vi "Transient Amb.vi"() -> ()   [LabVIEW 2015]
uses:
  <vilib>/Platform/TimedLoop/XDataNode/timing_clust.ctl
  <vilib>/Platform/TimedLoop/XDataNode/nitl_modes.ctl
  <vilib>/Platform/TimedLoop/XDataNode/wakeup.ctl
  <vilib>/DAQmx/read.llb/DAQmx Read (Analog DBL 1Chan 1Samp).vi
  <vilib>/DAQmx/read.llb/DAQmx Read (Analog 1D DBL NChan 1Samp).vi
  <vilib>/DAQmx/create/channels.llb/DAQmx Create Channel (AI-Voltage-Basic).vi
  <vilib>/DAQmx/miscellaneous.llb/DAQmx Fill In Error Info.vi
  <vilib>/Platform/TimedLoop/XDataNode/XDataNode.xnode
  Program Files/neMESYS_SDK/neMESYS LabVIEW Kit/neMESYS LabVIEW Integration Kit.lvlib
  <vilib>/Platform/TimedLoop/XDataNode/XDNodeRunTimeDep.lvlib
  Conor/Temp CN7500/Omega CN7500/Omega CN7500.lvlib
panel:
  out "Iteration Number":dbl
  in  "Ramp Temp":bool
  in  "Temp Decrease per Minute":dbl
  in  "Start Temp":dbl
  in  "Minutes at Start Conditions":dbl
  in  "Ramp Flow":bool
  in  "Flow Decrease per Minute":dbl
  in  "Start Flowrate":dbl
  in  "Flowrate 4":dbl
  in  "Flowrate 3":dbl
  in  "Flowrate 2":dbl
  in  "Flowrate 1":dbl
  in  "Temp Set Point":dbl
  out "Liquid Inlet Pressure (bar g)":dbl
  in  "Liquid P sensor Terminal Configuration":i32(ring)=-1 items=["default"=-1, "RSE"=10083, "NRSE"=10078, "Differential"=10106, "Pseudodifferential"=12529]
  in  "Liquid P sensor Physical Channel":tag="Dev1/ai0"
  in  "Safety or Emergency Syringe Control":bool
  out "Total Flowrate (uL/min)":dbl
  out "Gas Back Pressure (barg)":dbl
  in  "Shut down in empty?\nLeft off, right on":bool
  in  "Clear":bool
  out "Safety Shut Down Pressure (barg)":dbl
  out "Calculated Pressure":dbl[](graph)
  out "Safety Shut Down Temp":dbl
  out "Actual Temp (oC)":dbl
  out "Temperature":dynamicdata(graph)
  out "Temp Set Point (oC)":dbl
  in  "Stop everything":bool
  in  "Refill 4":bool
  in  "Refill 3":bool
  in  "Refill 2":bool
  in  "Refill 1":bool
  in  "Empty 4":bool
  in  "Empty 3":bool
  in  "Empty 2":bool
  in  "Empty 1":bool
  in  "Calibrate 4":bool
  in  "Calibrate 3":bool
  in  "Calibrate 2":bool
  in  "Calibrate 1":bool
  in  "Stop Dose 4":bool
  in  "Stop Dose 3":bool
  in  "Stop Dose 2":bool
  in  "Stop Dose 1":bool
  out "Syringe Level 4":dbl(slide) scale=0.0..5500.0
  out "Syringe Level 3":dbl(slide) scale=0.0..5500.0
  out "Syringe Level 2":dbl(slide) scale=0.0..5500.0
  out "Syringe Level 1":dbl(slide) scale=0.0..5500.0
  out "Flowrate 4 Ethanol":dbl
  out "Flowrate 3 Acid":dbl
  out "Flowrate 2 High":dbl
  out "Flowrate 1 Low":dbl
  # "Safety (start and end)"
  # "Current Conditions"
  # "(uL/min)"
  # "Coerced to nearest possible"
  # "If either ramps are off you need to manually enter the constant flowrate or temperature in the \nbottom sections"
  # "This code just uses 2 syringes\nThe ones at the right hand side"
  # "Emergency Syringe Control Below"
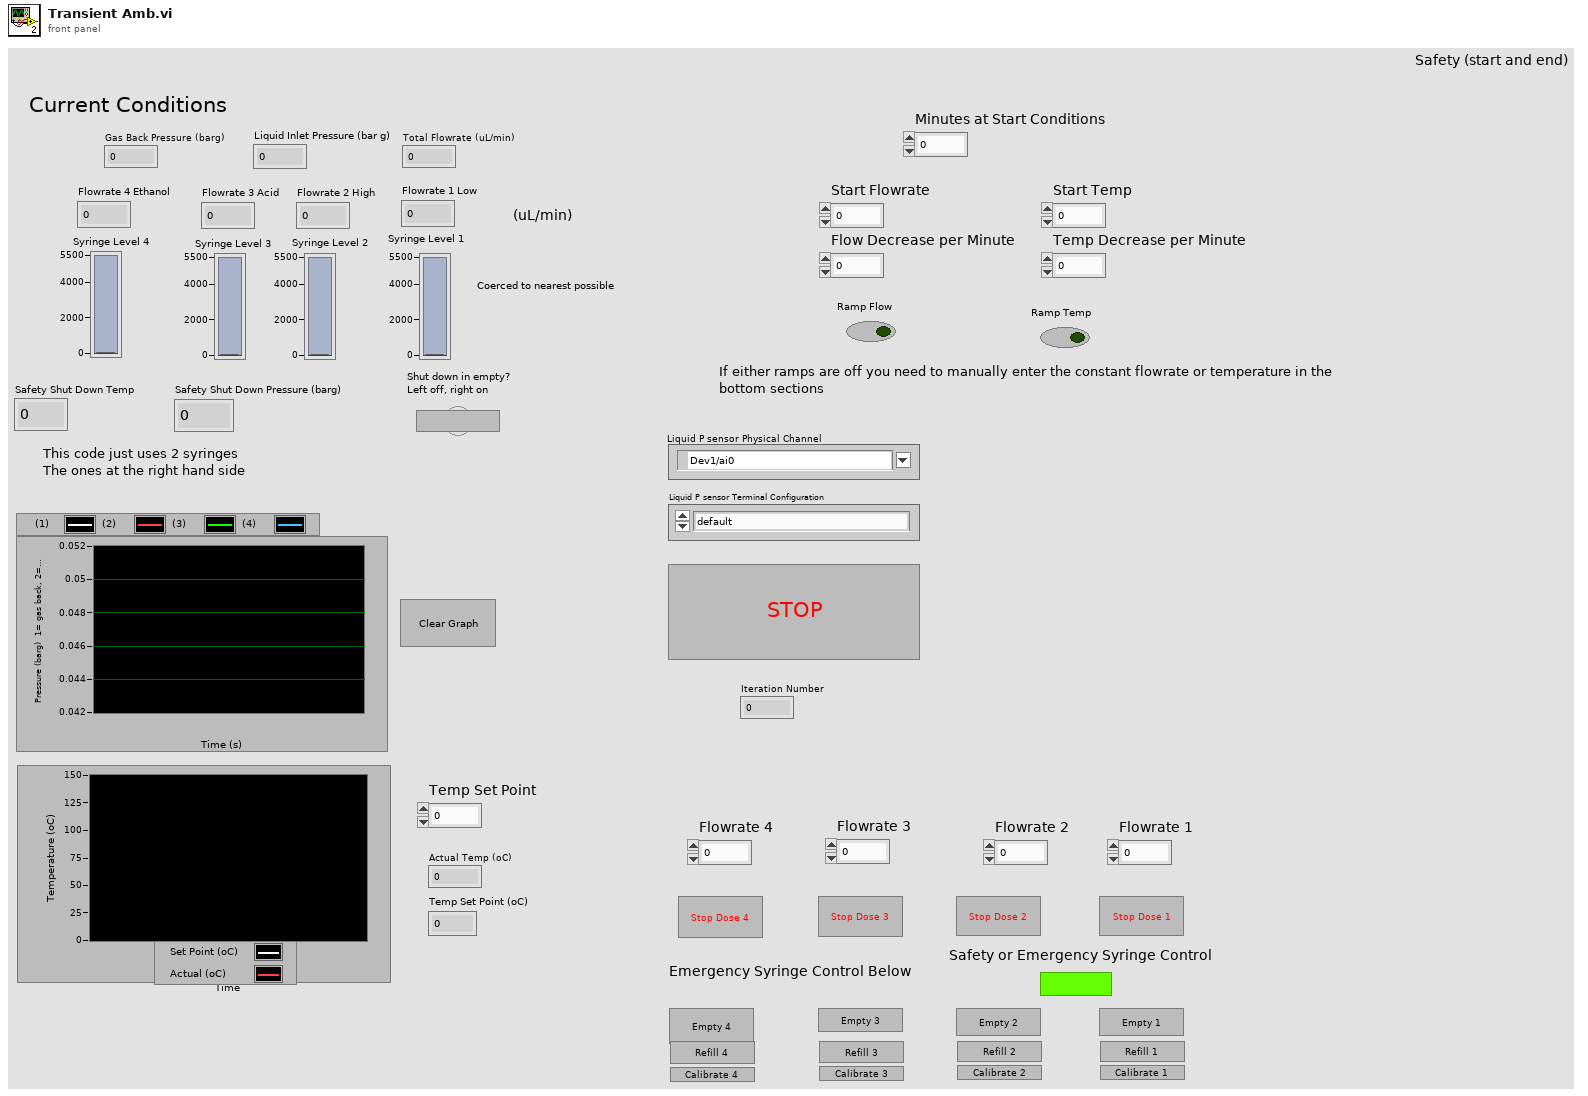
[diagram p1: front panel]
types:
  T1 = typedef "XDNodeRunTimeDep.lvlib/timing_clust.ctl" = cluster{"Expected End [f-1]":u64, "Actual End [f-1]":u64, "Finished Late? [f-1]":bool, "Expected End [i-1]":u64, "Actual End [i-1]":u64, "Finished Late? [i-1]":bool, "Expected Start [i]":u64, "Actual Start [i]":u64, "Expected Start [f]":u64, "Actual Start [f]":u64, "Source Name":string, "Structure Name":string, "Period":i64, "Deadline":i64, "Offset":i64, "Start":i64, "Priority":i32, "Timeout":i32, "Mode":T2, "Wakeup Reason":T3, "Error":errorcluster, "Source Type":string, "Secondary Source Type":string, "Global End Time":u64, "Global Start Time":u64, "Frame Duration":u64, "Iteration Duration":u64, "Assigned CPU":i32, "I/O Scan Engine Mode":u32}
  T2 = typedef "XDNodeRunTimeDep.lvlib/nitl_modes.ctl" = enum32{"No Change", "Process missed periods, maintain original phase", "Discard missed periods, maintain original phase", "Process missed periods, ignore original phase", "Discard missed periods, ignore original phase"}
  T3 = typedef "XDNodeRunTimeDep.lvlib/wakeup.ctl" = enum32{"Normal", "Aborted", "Asynchronous wakeup", "Timing source error", "Timed loop error", "Timeout"}
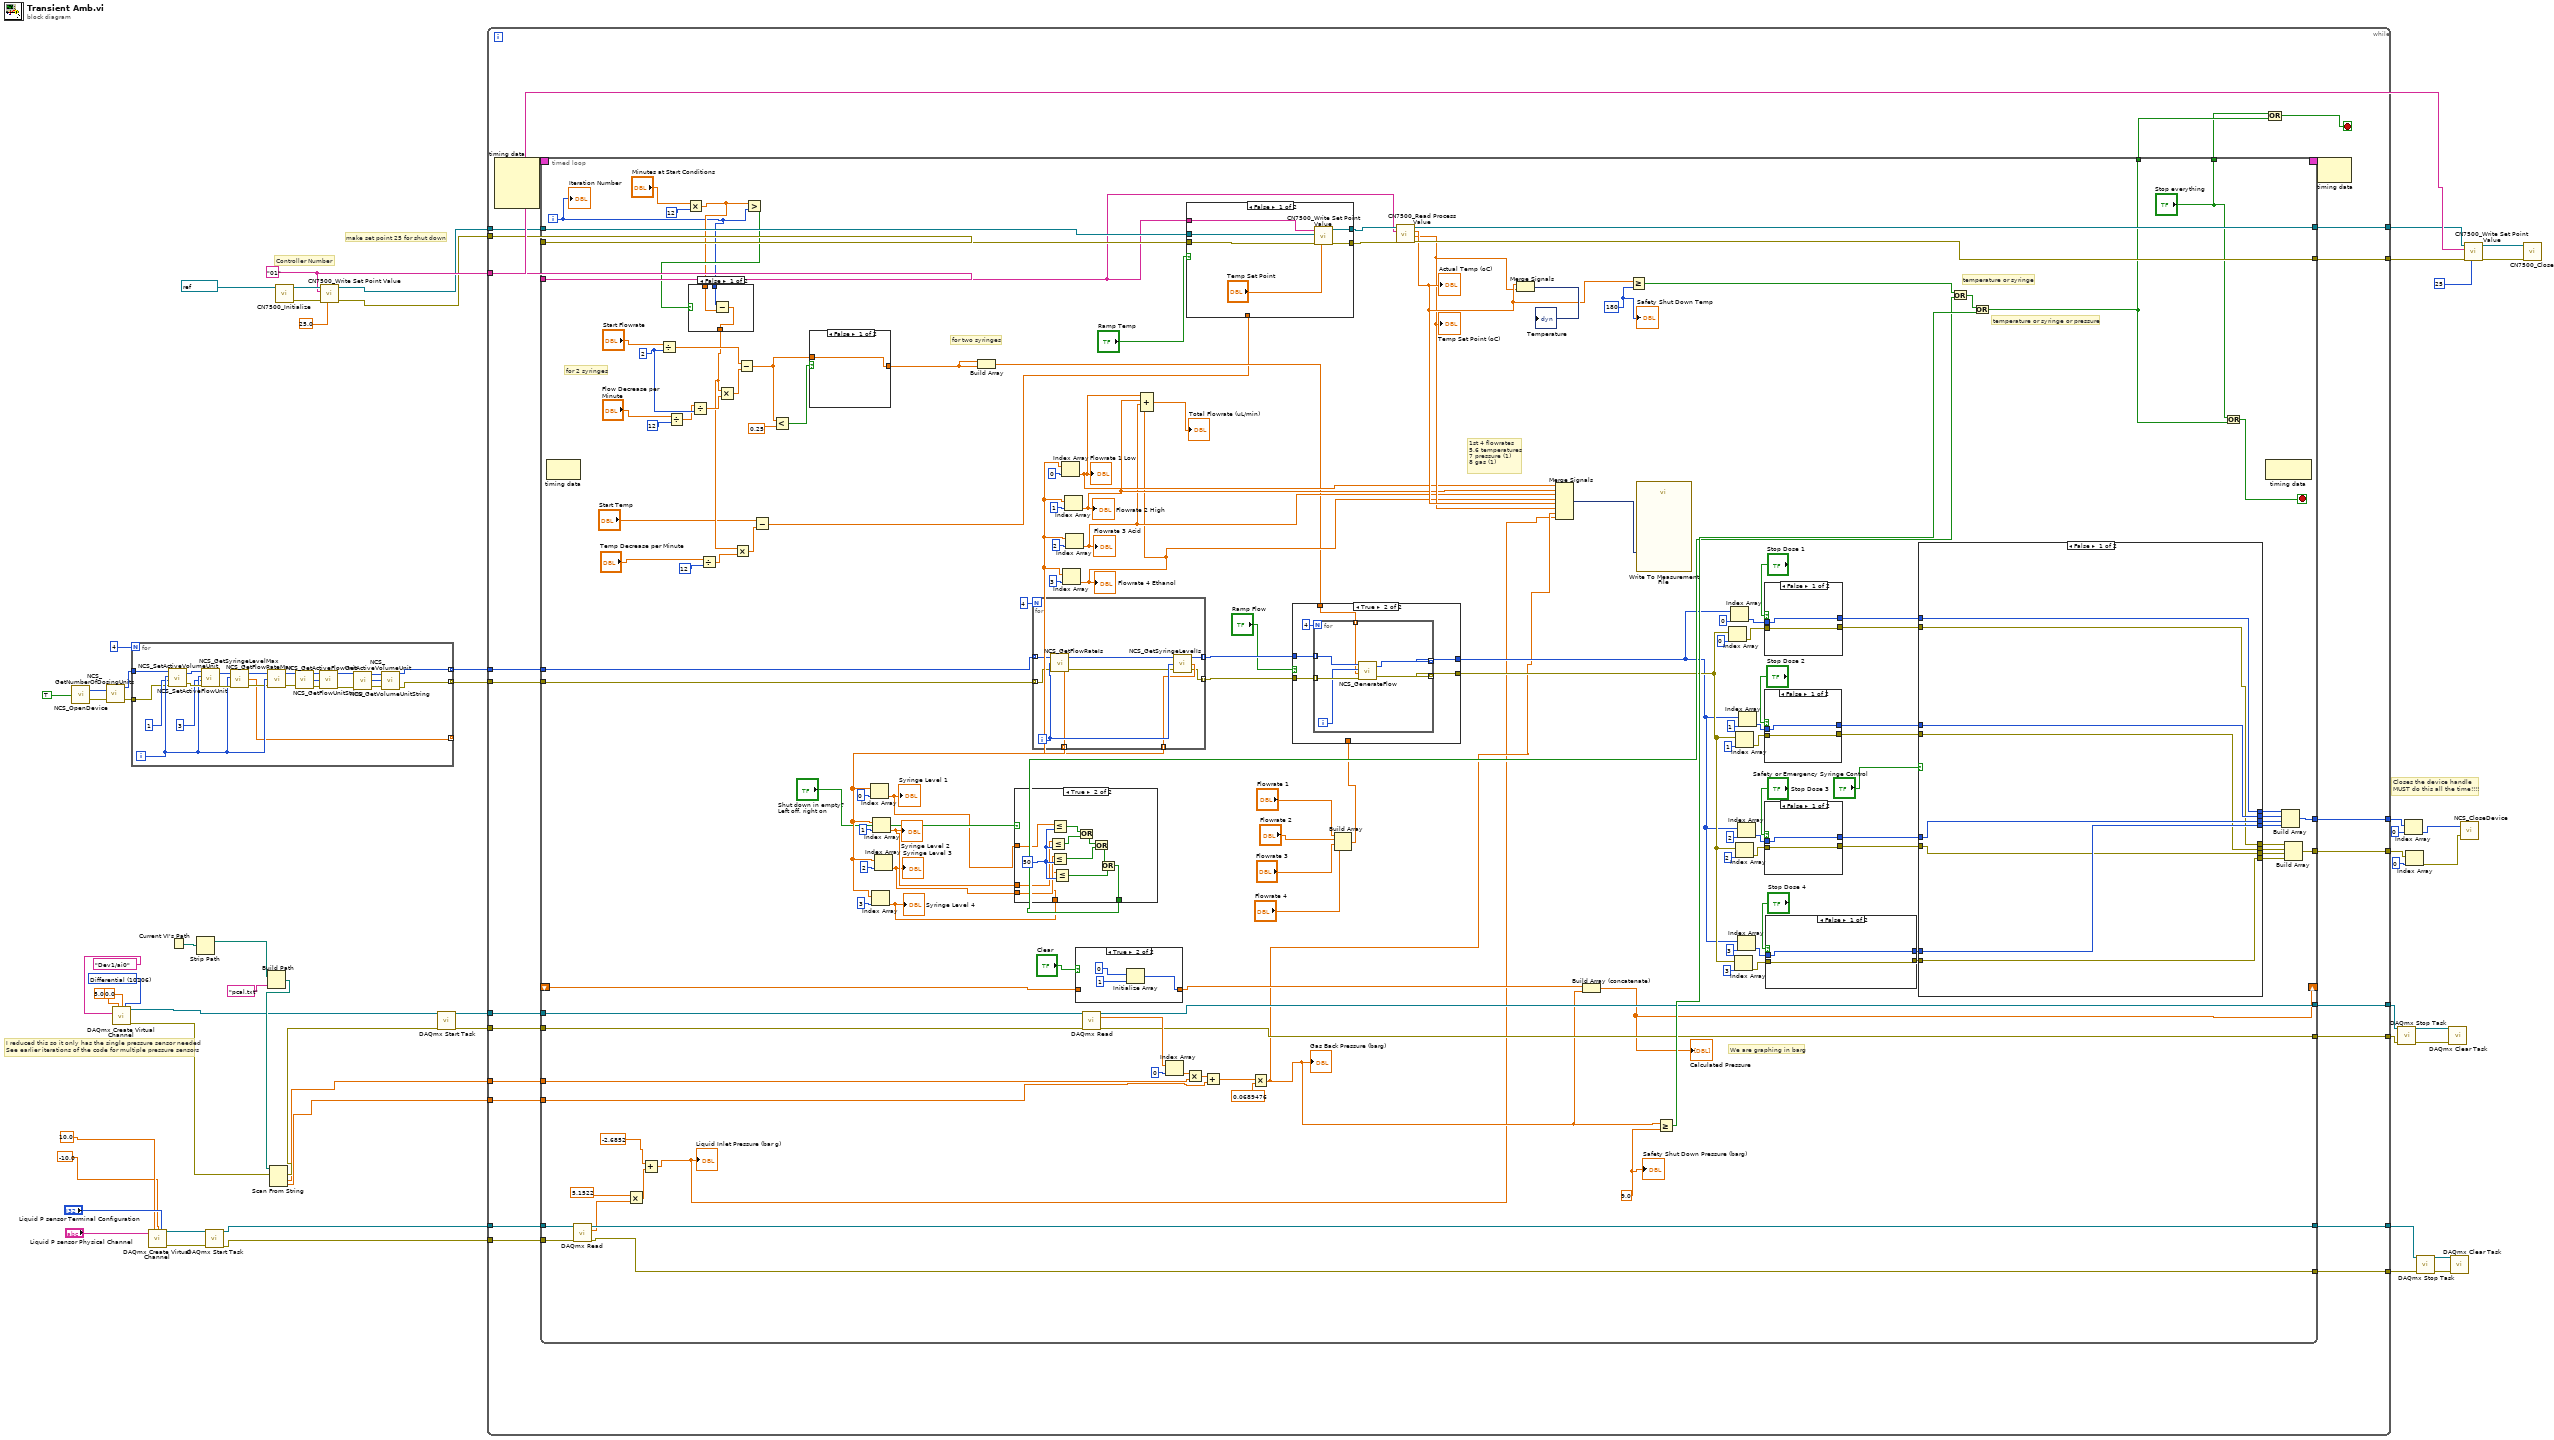
[diagram p0: block diagram]
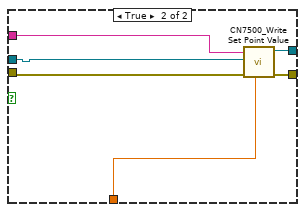
[diagram p2: hidden frame]
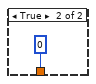
[diagram p3: hidden frame]
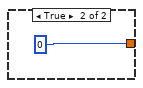
[diagram p4: hidden frame]
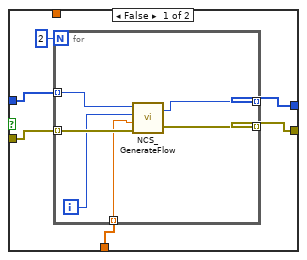
[diagram p5: hidden frame]
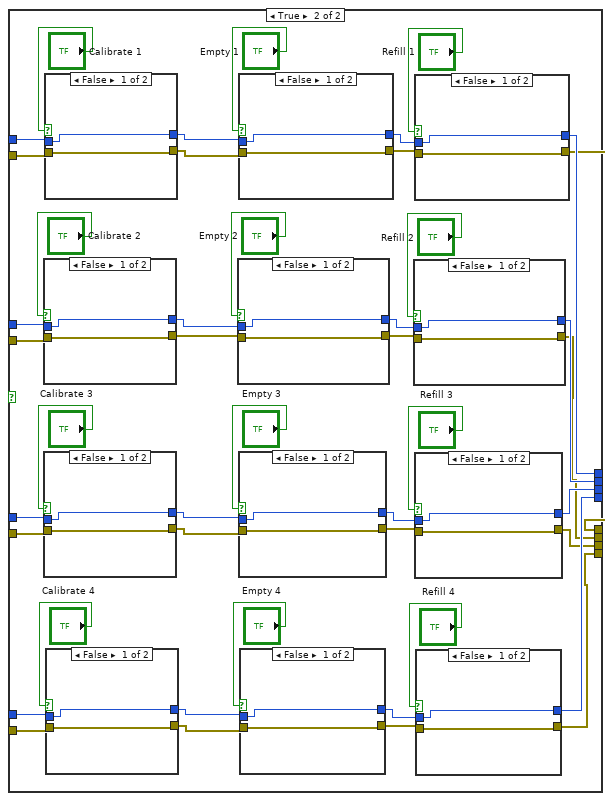
[diagram p6: hidden frame]
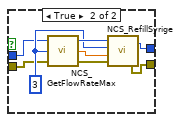
[diagram p7: hidden frame]
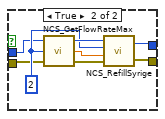
[diagram p8: hidden frame]
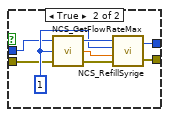
[diagram p9: hidden frame]
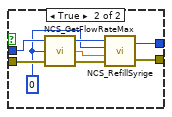
[diagram p10: hidden frame]
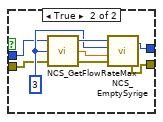
[diagram p11: hidden frame]
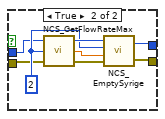
[diagram p12: hidden frame]
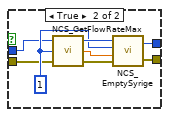
[diagram p13: hidden frame]
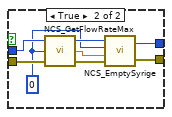
[diagram p14: hidden frame]
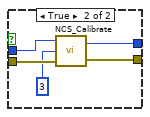
[diagram p15: hidden frame]
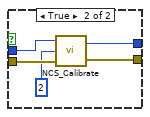
[diagram p16: hidden frame]
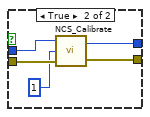
[diagram p17: hidden frame]
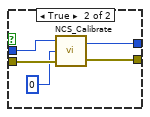
[diagram p18: hidden frame]
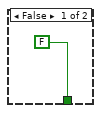
[diagram p19: hidden frame]
diagram:
  w29 = 10106 items=["default"=-1, "RSE"=10083, "NRSE"=10078, "Differential"=10106, "Pseudodifferential"=12529] ("input terminal configuration")
  w36 = "01" ("Controller Number")
  # "I reduced this so it only has the single pressure sensor needed\nSee earlier iterations of the code for multiple pressure sensors"
  # "make set point 25 for shut down"
  # "Controller Number"
  # "Closes the device handle \nMUST do this all the time!!!!"
  n1 = call "NCS_OpenDevice.vi"("show status window"=TRUE) -> ("device handle"=w55:u32, "error out"=w54:errorcluster)
  n2 = call "NCS_GetNumberOfDosingUnits.vi"("device handle in"=w55, "error in (no error)"=w54) -> ("device handle out"=w52:u32, "error out"=w53:errorcluster)  [unwired: 1 out]
  n3 = call-poly <vilib>:"DAQmx Create Virtual Channel.vi"("maximum value"=5.0, "minimum value"=0.0, "input terminal configuration"=w29, "physical channels"=tag "Dev1/ai0") -> ("task out"=w13:refnum<k21>, "error out"=w14:errorcluster)  [unwired: 10 in]
  n4 = for {
    N: 4 -> [_]
    tunnel: [w61] -> w51 mode=indexing
    tunnel: [w60] -> w50 mode=indexing
    tunnel: [w74] -> _ mode=indexing
    tunnel: w53 -> [w59]
    tunnel: w52 -> [w58]
    i -> [w77]
    n5 = call "NCS_SetActiveVolumeUnit.vi"("error in (no error)"=w59, "active volume unit"=1, "dosingunit"=w77, "device handle in"=w58) -> ("error out"=w80:errorcluster, "device handle out"=w81:u32)
    n6 = call "NCS_SetActiveFlowUnit.vi"("error in (no error)"=w80, "active flow unit"=3, "dosingunit"=w77, "device handle in"=w81) -> ("error out"=w78:errorcluster, "device handle out"=w79:u32)
    n7 = call "NCS_GetSyringeLevelMax.vi"("error in (no error)"=w78, "dosingunit"=w77, "device handle in"=w79) -> ("error out"=w75:errorcluster, "syringe level max"=w74:dbl, "device handle out"=w76:u32)  [unwired: 1 out]
    n8 = call "NCS_GetFlowRateMax.vi"("error in (no error)"=w75, "dosingunit"=w77, "device handle in"=w76) -> ("error out"=w62:errorcluster, "device handle out"=w63:u32)  [unwired: 1 out]
    n9 = call "NCS_GetActiveFlowUnit.vi"("error in (no error)"=w62, "device handle in"=w63) -> ("error out"=w70:errorcluster, "active flow unit"=w69:u8, "device handle out"=w71:u32)  [unwired: 1 in]
    n10 = call "NCS_GetFlowUnitString.vi"("device handle in"=w71, "flow unit id"=w69, "error in (no error)"=w70) -> ("device handle out"=w66:u32, "error out"=w65:errorcluster)  [unwired: 2 out]
    n11 = call "NCS_GetActiveVolumeUnit.vi"("error in (no error)"=w65, "device handle in"=w66) -> ("error out"=w67:errorcluster, "active volume unit"=w68:u8, "device handle out"=w64:u32)  [unwired: 1 in]
    n12 = call "NCS_GetVolumeUnitString.vi"("device handle in"=w64, "volume unit id"=w68, "error in (no error)"=w67) -> ("device handle out"=w61:u32, "error out"=w60:errorcluster)  [unwired: 2 out]
  }
  n13 = call-poly <vilib>:"DAQmx Create Virtual Channel.vi"("maximum value"=10.0, "minimum value"=-10.0 ("maximum value"), "input terminal configuration"="Liquid P sensor Terminal Configuration", "physical channels"="Liquid P sensor Physical Channel") -> ("task out"=w9:refnum<k21>, "error out"=w10:errorcluster)  [unwired: 10 in]
  n14 = Current VI's Path() -> (path=w27:path)
  n15 = Strip Path(path=w27) -> (stripped path=w25:path)  [unwired: 1 out]
  n16 = call <vilib>:"DAQmx Start Task.vi"("task/channels in"=w9, "error in"=w10) -> ("task out"=w8:refnum<k21>, "error out"=w7:errorcluster)  [unwired: 12 in]
  n17 = Build Path(base path=w25, name or relative path="pcal.txt") -> (appended path=w26:path)
  n18 = Scan From String(w26, w14) -> (w23:errorcluster, output 1=w20:dbl, output 2=w19:dbl)  [unwired: 3 in, 1 out]
  n19 = call "CN7500_Initialize.vi"("VISA resource name"=refnum<visa-resource-name> "COM8") -> ("error out"=w42:errorcluster, "VISA resource name out"=w43:refnum<visa-resource-name>)  [unwired: 9 in]
  n20 = call "CN7500_Write Set Point Value.vi"("Target Set Point Value"=25.0, "error in (no error)"=w42, "Controller Number"=w36, "VISA In"=w43) -> ("error out"=w34:errorcluster, "VISA Out"=w35:refnum<visa-resource-name>)  [unwired: 6 in]
  n21 = call <vilib>:"DAQmx Start Task.vi"("task/channels in"=w13, "error in"=w23) -> ("task out"=w22:refnum<k21>, "error out"=w21:errorcluster)  [unwired: 12 in]
  n22 = while {
    tunnel: w51 -> [w105]
    tunnel: w50 -> [w104]
    tunnel: [w103] -> w45
    tunnel: [w102] -> w44
    tunnel: w36 -> [w99]
    tunnel: w35 -> [w98]
    tunnel: w34 -> [w97]
    tunnel: [w96] -> w33
    tunnel: [w95] -> w32
    tunnel: w22 -> [w93]
    tunnel: w21 -> [w92]
    tunnel: w20 -> [w91]
    tunnel: w19 -> [w90]
    tunnel: [w89] -> w16
    tunnel: [w88] -> w15
    tunnel: w8 -> [w85]
    tunnel: w7 -> [w84]
    tunnel: [w83] -> w5
    tunnel: [w82] -> w3
    stop <- w87 stop-if-true
    n23 = node-c288() -> (w101:T1)  [unwired: 4 in]
    n24 = timed-loop {
      tunnel: w105 -> [w248]
      tunnel: w104 -> [w247]
      tunnel: [w198] -> w103
      tunnel: [w197] -> w102
      timing: w101 -> [_]
      timing-out: [_] -> w100
      tunnel: w99 -> [w191]
      tunnel: w98 -> [w195]
      tunnel: w97 -> [w194]
      tunnel: [w190] -> w96
      tunnel: [w189] -> w95
      tunnel: [w133] -> w94
      tunnel: w93 -> [w177]
      tunnel: w92 -> [w176]
      tunnel: w91 -> [w175]
      tunnel: w90 -> [w174]
      shift-right: [w154] -> _
      shift-left: _ -> [w167]
      tunnel: [w170] -> w89
      tunnel: [w169] -> w88
      tunnel: ["Stop everything"] -> w86
      tunnel: w85 -> [w153]
      tunnel: w84 -> [w152]
      tunnel: [w151] -> w83
      tunnel: [w150] -> w82
      i -> [w106]
      stop <- w165 stop-if-true
      w121 = 2
      w173 = 9.0 ("Safety Shut Down Pressure (barg)")
      w187 = 180
      # "for two syringes"
      # "for 2 syringes"
      # "1st 4 flowrates\n5,6 temperatures\n7 pressure (1)\n8 gas (1)"
      # "temperature or syringe or pressure"
      # "We are graphing in barg"
      # "temperature or syringe"
      n25 = node-c288() -> ()  [unwired: 1 in, 1 out]
      n26 = call-poly <vilib>:"DAQmx Read.vi"("task/channels in"=w153, "error in"=w152) -> ("task out"=w151:refnum<k21>, "data"=w146:dbl, "error out"=w150:errorcluster)  [unwired: 11 in]
      n27 = Multiply(x=5.1522, y=w146) -> (x*y=w149:dbl)
      n28 = Add(x=-2.6852, y=w149) -> (x+y=w144:dbl)
      "Liquid Inlet Pressure (bar g)" <- w144
      n29 = Divide(x="Start Flowrate", y=w121) -> (x/y=w129:dbl)
      n30 = Divide(x="Flow Decrease per Minute", y=12) -> (x/y=w120:dbl)
      n31 = Multiply(x="Minutes at Start Conditions", y=12) -> (x*y=w115:dbl)
      n32 = Divide(x=w120, y=w121) -> (x/y=w119:dbl)
      n33 = Divide(x="Temp Decrease per Minute", y=12) -> (x/y=w111:dbl)
      n34 = Greater?(x=w115, y=w106) -> (0:w116:bool)
      n35 = case shown="False" w116 {
        tunnel: [w262 0] -> w110
        tunnel: w106 -> [w264 _]
        tunnel: w115 -> [w263 _]
        frame False {
          n36 = Subtract(x=w264, y=w263) -> (x-y=w262:dbl)
        }
        frame True {
        }
      }
      n37 = Multiply(x=w110, y=w119) -> (x*y=w128:dbl)
      n38 = Multiply(x=w110, y=w111) -> (x*y=w112:dbl)
      n39 = Subtract(x=w129, y=w128) -> (x-y=w122:dbl)
      n40 = Subtract(x="Start Temp", y=w112) -> (x-y=w107:dbl)
      n41 = Less?(x=w122, y=0.25) -> (x < y?=w124:bool)
      n42 = case shown="False" w124 {
        tunnel: [w266 0] -> w123
        tunnel: w122 -> [w266 _]
        frame False {
        }
        frame True {
        }
      }
      n43 = Build Array(w123, w123) -> (w126:dbl[])
      n44 = for {
        N: 4 -> [_]
        tunnel: w248 -> [w507] mode=indexing
        tunnel: [w505] -> w242 mode=indexing
        tunnel: [w502] -> w237 mode=indexing
        tunnel: [w501] -> w236 mode=indexing
        tunnel: [w500] -> w235 mode=indexing
        tunnel: w247 -> [w499] mode=indexing
        i -> [w506]
        n45 = call "NCS_GetFlowRateIs.vi"("error in (no error)"=w499, "dosingunit"=w506, "device handle in"=w507) -> ("error out"=w503:errorcluster, "flowrate is"=w505:dbl, "device handle out"=w504:u32)
        n46 = call "NCS_GetSyringeLevelIs.vi"("error in (no error)"=w503, "dosingunit"=w506, "device handle in"=w504) -> ("error out"=w500:errorcluster, "syringe level is"=w502:dbl, "device handle out"=w501:u32)
      }
      n47 = Index Array(array=w237, index=0) -> (element=w162:dbl)
      "Syringe Level 1" <- w162
      n48 = Index Array(array=w237, index=3) -> (element=w159:dbl)
      "Syringe Level 4" <- w159
      n49 = Index Array(array=w237, index=1) -> (element=w161:dbl)
      "Syringe Level 2" <- w161
      n50 = Index Array(array=w237, index=2) -> (element=w160:dbl)
      "Syringe Level 3" <- w160
      n51 = case shown="True" "Shut down in empty?\nLeft off, right on" {
        tunnel: [FALSE w457] -> w163
        tunnel: w162 -> [_ w456]
        tunnel: w161 -> [_ w455]
        tunnel: w160 -> [_ w454]
        tunnel: w159 -> [_ w453]
        frame False {
        }
        frame True {
          w458 = 50
          n52 = Less Or Equal?(x=w455, y=w458) -> (x <= y?=w464:bool)
          n53 = Less Or Equal?(x=w456, y=w458) -> (x <= y?=w459:bool)
          n54 = Less Or Equal?(x=w454, y=w458) -> (x <= y?=w462:bool)
          n55 = Less Or Equal?(x=w453, y=w458) -> (x <= y?=w460:bool)
          n56 = Or(x=w459, y=w464) -> (x .or. y?=w463:bool)
          n57 = Or(x=w463, y=w462) -> (x .or. y?=w461:bool)
          n58 = Or(x=w461, y=w460) -> (x .or. y?=w457:bool)
        }
      }
      n59 = Index Array(array=w242, index=0) -> (element=w142:dbl)
      "Flowrate 1 Low" <- w142
      n60 = Index Array(array=w242, index=3) -> (element=w139:dbl)
      "Flowrate 4 Ethanol" <- w139
      n61 = Index Array(array=w242, index=1) -> (element=w141:dbl)
      "Flowrate 2 High" <- w141
      n62 = Index Array(array=w242, index=2) -> (element=w140:dbl)
      "Flowrate 3 Acid" <- w140
      n63 = case shown="True" "Clear" {
        tunnel: w167 -> [w465 _]
        tunnel: [w465 w466] -> w166
        frame False {
        }
        frame True {
          n64 = Initialize Array(0, 1) -> (w466:i32[])
        }
      }
      n65 = call-poly <vilib>:"DAQmx Read.vi"("task/channels in"=w177, "error in"=w176) -> ("task out"=w170:refnum<k21>, "data"=w182:dbl[], "error out"=w169:errorcluster)  [unwired: 11 in]
      n66 = Compound Arithmetic op=ADD(w142, w141, w140, w139) -> (→"Total Flowrate (uL/min)":dbl)
      n67 = Index Array(array=w182, index=0) -> (element=w180:dbl)
      n68 = Multiply(x=w180, y=w175) -> (x*y=w181:dbl)
      n69 = case shown="False" "Ramp Temp" {
        tunnel: w195 -> [w255 w260]
        tunnel: w194 -> [w254 w259]
        tunnel: [w253 w258] -> w193
        tunnel: [w252 w257] -> w192
        tunnel: w191 -> [w251 w261]
        tunnel: w107 -> [_ w256]
        frame False {
          n70 = call "CN7500_Write Set Point Value.vi"("Target Set Point Value"="Temp Set Point", "error in (no error)"=w254, "Controller Number"=w251, "VISA In"=w255) -> ("error out"=w252:errorcluster, "VISA Out"=w253:refnum<visa-resource-name>)  [unwired: 6 in]
        }
        frame True {
          n71 = call "CN7500_Write Set Point Value.vi"("Target Set Point Value"=w256, "error in (no error)"=w259, "Controller Number"=w261, "VISA In"=w260) -> ("error out"=w257:errorcluster, "VISA Out"=w258:refnum<visa-resource-name>)  [unwired: 6 in]
        }
      }
      n72 = Add(x=w181, y=w174) -> (x+y=w178:dbl)
      n73 = Multiply(x=w178, y=0.0689476) -> (x*y=w145:dbl)
      "Gas Back Pressure (barg)" <- w145
      n74 = Build Array("Flowrate 1", "Flowrate 2", "Flowrate 3", "Flowrate 4") -> (w134:dbl[])
      n75 = case shown="True" "Ramp Flow" {
        tunnel: w236 -> [w272 w285]
        tunnel: w235 -> [w271 w284]
        tunnel: [w269 w283] -> w157
        tunnel: [w268 w282] -> w156
        tunnel: w134 -> [w270 _]
        tunnel: w126 -> [_ w280]
        frame False {
          n76 = for {
            N: 2 -> [_]
            tunnel: w272 -> [w279] mode=indexing
            tunnel: w271 -> [w278] mode=indexing
            tunnel: [w277] -> w269 mode=indexing
            tunnel: [w276] -> w268 mode=indexing
            tunnel: w270 -> [w274] mode=indexing
            i -> [w275]
            n77 = call "NCS_GenerateFlow.vi"("error in (no error)"=w278, "flowrate"=w274, "dosingunit"=w275, "device handle in"=w279) -> ("error out"=w277:errorcluster, "device handle out"=w276:u32)
          }
        }
        frame True {
          n78 = for {
            N: 4 -> [_]
            tunnel: w285 -> [w291] mode=indexing
            tunnel: w284 -> [w290] mode=indexing
            tunnel: [w289] -> w283 mode=indexing
            tunnel: [w288] -> w282 mode=indexing
            tunnel: w280 -> [w286] mode=indexing
            i -> [w287]
            n79 = call "NCS_GenerateFlow.vi"("error in (no error)"=w290, "flowrate"=w286, "dosingunit"=w287, "device handle in"=w291) -> ("error out"=w289:errorcluster, "device handle out"=w288:u32)
          }
        }
      }
      n80 = call "CN7500_Read Process Value.vi"("error in (no error)"=w192, "Controller Number"=w191, "VISA In"=w193) -> ("error out"=w190:errorcluster, "Set Point Value"=w184:dbl, "Process Value"=w185:dbl, "VISA Out"=w189:refnum<visa-resource-name>)  [unwired: 5 in]
      "Temp Set Point (oC)" <- w184
      "Actual Temp (oC)" <- w185
      n81 = Merge Signals(w185, w184) -> (→"Temperature":dynamicdata)
      n82 = Merge Signals(w142, w141, w140, w139, w185, w184, w145, w144) -> (w196:dynamicdata)
      n83 = Build Array (concatenate)(w166, w145) -> (w154:dbl[])
      "Calculated Pressure" <- w154
      n84 = Greater Or Equal?(x=w185, y=w187) -> (x >= y?=w186:bool)
      n85 = call "Write To Measurement File"("Signals"=w196) -> ()  [unwired: 16 in, 3 out]
      n86 = Greater Or Equal?(x=w145, y=w173) -> (x >= y?=w171:bool)
      n87 = Index Array(array=w157, index=0) -> (element=w225:errorcluster)
      n88 = Index Array(array=w156, index=0) -> (element=w226:u32)
      n89 = Index Array(array=w157, index=3) -> (element=w215:errorcluster)
      n90 = Index Array(array=w157, index=2) -> (element=w217:errorcluster)
      n91 = Index Array(array=w157, index=1) -> (element=w219:errorcluster)
      n92 = Index Array(array=w156, index=3) -> (element=w216:u32)
      n93 = Index Array(array=w156, index=2) -> (element=w218:u32)
      n94 = Index Array(array=w156, index=1) -> (element=w220:u32)
      n95 = case shown="False" "Stop Dose 2" {
        tunnel: w220 -> [w486 w491]
        tunnel: w219 -> [w485 w490]
        tunnel: [w486 w489] -> w212
        tunnel: [w485 w488] -> w211
        frame False {
        }
        frame True {
          n96 = call "NCS_Stop.vi"("error in (no error)"=w490, "dosingunit"=1, "device handle in"=w491) -> ("error out"=w488:errorcluster, "device handle out"=w489:u32)
        }
      }
      n97 = case shown="False" "Stop Dose 1" {
        tunnel: w226 -> [w493 w498]
        tunnel: w225 -> [w492 w497]
        tunnel: [w493 w496] -> w214
        tunnel: [w492 w495] -> w213
        frame False {
        }
        frame True {
          n98 = call "NCS_Stop.vi"("error in (no error)"=w497, "dosingunit"=0, "device handle in"=w498) -> ("error out"=w495:errorcluster, "device handle out"=w496:u32)
        }
      }
      n99 = case shown="False" "Stop Dose 3" {
        tunnel: w218 -> [w479 w484]
        tunnel: w217 -> [w478 w483]
        tunnel: [w479 w482] -> w210
        tunnel: [w478 w481] -> w209
        frame False {
        }
        frame True {
          n100 = call "NCS_Stop.vi"("error in (no error)"=w483, "dosingunit"=2, "device handle in"=w484) -> ("error out"=w481:errorcluster, "device handle out"=w482:u32)
        }
      }
      n101 = case shown="False" "Stop Dose 4" {
        tunnel: w216 -> [w472 w477]
        tunnel: w215 -> [w471 w476]
        tunnel: [w472 w475] -> w208
        tunnel: [w471 w474] -> w207
        frame False {
        }
        frame True {
          n102 = call "NCS_Stop.vi"("error in (no error)"=w476, "dosingunit"=3, "device handle in"=w477) -> ("error out"=w474:errorcluster, "device handle out"=w475:u32)
        }
      }
      n103 = case shown="False" "Safety or Emergency Syringe Control" {
        tunnel: w214 -> [w299 w340]
        tunnel: w213 -> [w295 w339]
        tunnel: w212 -> [w298 w338]
        tunnel: w211 -> [w294 w337]
        tunnel: w210 -> [w297 w336]
        tunnel: w209 -> [w293 w335]
        tunnel: w208 -> [w296 w334]
        tunnel: w207 -> [w292 w333]
        tunnel: [w299 w310] -> w206
        tunnel: [w298 w309] -> w205
        tunnel: [w297 w308] -> w204
        tunnel: [w296 w307] -> w203
        tunnel: [w294 w306] -> w202
        tunnel: [w293 w305] -> w201
        tunnel: [w292 w304] -> w200
        tunnel: [w295 w300] -> w199
        frame False {
        }
        frame True {
          n104 = case shown="False" "Calibrate 2" {
            tunnel: w338 -> [w439 w444]
            tunnel: w337 -> [w438 w443]
            tunnel: [w439 w442] -> w327
            tunnel: [w438 w441] -> w326
            frame False {
            }
            frame True {
              n105 = call "NCS_Calibrate.vi"("error in (no error)"=w443, "dosingunit"=1, "device handle in"=w444) -> ("error out"=w441:errorcluster, "device handle out"=w442:u32)
            }
          }
          n106 = case shown="False" "Calibrate 3" {
            tunnel: w336 -> [w432 w437]
            tunnel: w335 -> [w431 w436]
            tunnel: [w432 w435] -> w325
            tunnel: [w431 w434] -> w324
            frame False {
            }
            frame True {
              n107 = call "NCS_Calibrate.vi"("error in (no error)"=w436, "dosingunit"=2, "device handle in"=w437) -> ("error out"=w434:errorcluster, "device handle out"=w435:u32)
            }
          }
          n108 = case shown="False" "Calibrate 1" {
            tunnel: w340 -> [w446 w451]
            tunnel: w339 -> [w445 w450]
            tunnel: [w446 w449] -> w329
            tunnel: [w445 w448] -> w328
            frame False {
            }
            frame True {
              n109 = call "NCS_Calibrate.vi"("error in (no error)"=w450, "dosingunit"=0, "device handle in"=w451) -> ("error out"=w448:errorcluster, "device handle out"=w449:u32)
            }
          }
          n110 = case shown="False" "Calibrate 4" {
            tunnel: w334 -> [w425 w430]
            tunnel: w333 -> [w424 w429]
            tunnel: [w425 w428] -> w323
            tunnel: [w424 w427] -> w322
            frame False {
            }
            frame True {
              n111 = call "NCS_Calibrate.vi"("error in (no error)"=w429, "dosingunit"=3, "device handle in"=w430) -> ("error out"=w427:errorcluster, "device handle out"=w428:u32)
            }
          }
          n112 = case shown="False" "Empty 2" {
            tunnel: w327 -> [w405 w409]
            tunnel: w326 -> [w404 w407]
            tunnel: [w405 w408] -> w313
            tunnel: [w404 w406] -> w314
            frame False {
            }
            frame True {
              w411 = 1
              n113 = call "NCS_GetFlowRateMax.vi"("error in (no error)"=w407, "dosingunit"=w411, "device handle in"=w409) -> ("error out"=w412:errorcluster, "flow rate max"=w410:dbl, "device handle out"=w413:u32)
              n114 = call "NCS_EmptySyrige.vi"("error in (no error)"=w412, "flowrate"=w410, "dosingunit"=w411, "device handle in"=w413) -> ("error out"=w406:errorcluster, "device handle out"=w408:u32)
            }
          }
          n115 = case shown="False" "Empty 1" {
            tunnel: w329 -> [w415 w423]
            tunnel: w328 -> [w414 w420]
            tunnel: [w415 w421] -> w311
            tunnel: [w414 w418] -> w312
            frame False {
            }
            frame True {
              w417 = 0
              n116 = call "NCS_GetFlowRateMax.vi"("error in (no error)"=w420, "dosingunit"=w417, "device handle in"=w423) -> ("error out"=w419:errorcluster, "flow rate max"=w416:dbl, "device handle out"=w422:u32)
              n117 = call "NCS_EmptySyrige.vi"("error in (no error)"=w419, "flowrate"=w416, "dosingunit"=w417, "device handle in"=w422) -> ("error out"=w418:errorcluster, "device handle out"=w421:u32)
            }
          }
          n118 = case shown="False" "Empty 3" {
            tunnel: w325 -> [w395 w396]
            tunnel: w324 -> [w394 w397]
            tunnel: [w395 w398] -> w315
            tunnel: [w394 w399] -> w316
            frame False {
            }
            frame True {
              w401 = 2
              n119 = call "NCS_GetFlowRateMax.vi"("error in (no error)"=w397, "dosingunit"=w401, "device handle in"=w396) -> ("error out"=w402:errorcluster, "flow rate max"=w400:dbl, "device handle out"=w403:u32)
              n120 = call "NCS_EmptySyrige.vi"("error in (no error)"=w402, "flowrate"=w400, "dosingunit"=w401, "device handle in"=w403) -> ("error out"=w399:errorcluster, "device handle out"=w398:u32)
            }
          }
          n121 = case shown="False" "Empty 4" {
            tunnel: w323 -> [w385 w386]
            tunnel: w322 -> [w384 w387]
            tunnel: [w385 w389] -> w317
            tunnel: [w384 w388] -> w318
            frame False {
            }
            frame True {
              w391 = 3
              n122 = call "NCS_GetFlowRateMax.vi"("error in (no error)"=w387, "dosingunit"=w391, "device handle in"=w386) -> ("error out"=w392:errorcluster, "flow rate max"=w390:dbl, "device handle out"=w393:u32)
              n123 = call "NCS_EmptySyrige.vi"("error in (no error)"=w392, "flowrate"=w390, "dosingunit"=w391, "device handle in"=w393) -> ("error out"=w388:errorcluster, "device handle out"=w389:u32)
            }
          }
          n124 = case shown="False" "Refill 2" {
            tunnel: w313 -> [w365 w369]
            tunnel: w314 -> [w364 w367]
            tunnel: [w365 w368] -> w309
            tunnel: [w364 w366] -> w306
            frame False {
            }
            frame True {
              w371 = 1
              n125 = call "NCS_GetFlowRateMax.vi"("error in (no error)"=w367, "dosingunit"=w371, "device handle in"=w369) -> ("error out"=w372:errorcluster, "flow rate max"=w370:dbl, "device handle out"=w373:u32)
              n126 = call "NCS_RefillSyrige.vi"("error in (no error)"=w372, "flowrate"=w370, "dosingunit"=w371, "device handle in"=w373) -> ("error out"=w366:errorcluster, "device handle out"=w368:u32)
            }
          }
          n127 = case shown="False" "Refill 1" {
            tunnel: w311 -> [w375 w383]
            tunnel: w312 -> [w374 w380]
            tunnel: [w375 w381] -> w310
            tunnel: [w374 w378] -> w300
            frame False {
            }
            frame True {
              w377 = 0
              n128 = call "NCS_GetFlowRateMax.vi"("error in (no error)"=w380, "dosingunit"=w377, "device handle in"=w383) -> ("error out"=w379:errorcluster, "flow rate max"=w376:dbl, "device handle out"=w382:u32)
              n129 = call "NCS_RefillSyrige.vi"("error in (no error)"=w379, "flowrate"=w376, "dosingunit"=w377, "device handle in"=w382) -> ("error out"=w378:errorcluster, "device handle out"=w381:u32)
            }
          }
          n130 = case shown="False" "Refill 3" {
            tunnel: w315 -> [w355 w356]
            tunnel: w316 -> [w354 w357]
            tunnel: [w355 w358] -> w308
            tunnel: [w354 w359] -> w305
            frame False {
            }
            frame True {
              w361 = 2
              n131 = call "NCS_GetFlowRateMax.vi"("error in (no error)"=w357, "dosingunit"=w361, "device handle in"=w356) -> ("error out"=w362:errorcluster, "flow rate max"=w360:dbl, "device handle out"=w363:u32)
              n132 = call "NCS_RefillSyrige.vi"("error in (no error)"=w362, "flowrate"=w360, "dosingunit"=w361, "device handle in"=w363) -> ("error out"=w359:errorcluster, "device handle out"=w358:u32)
            }
          }
          n133 = case shown="False" "Refill 4" {
            tunnel: w317 -> [w345 w346]
            tunnel: w318 -> [w344 w347]
            tunnel: [w345 w349] -> w307
            tunnel: [w344 w348] -> w304
            frame False {
            }
            frame True {
              w351 = 3
              n134 = call "NCS_GetFlowRateMax.vi"("error in (no error)"=w347, "dosingunit"=w351, "device handle in"=w346) -> ("error out"=w352:errorcluster, "flow rate max"=w350:dbl, "device handle out"=w353:u32)
              n135 = call "NCS_RefillSyrige.vi"("error in (no error)"=w352, "flowrate"=w350, "dosingunit"=w351, "device handle in"=w353) -> ("error out"=w348:errorcluster, "device handle out"=w349:u32)
            }
          }
        }
      }
      n136 = Or(x=w186, y=w163) -> (x .or. y?=w172:bool)
      n137 = Or(x=w172, y=w171) -> (x .or. y?=w133:bool)
      n138 = Or(x="Stop everything", y=w133) -> (x .or. y?=w165:bool)
      n139 = node-c288() -> ()  [unwired: 1 in, 1 out]
      n140 = Build Array(w206, w205, w204, w203) -> (w198:u32[])
      n141 = Build Array(w199, w202, w201, w200) -> (w197:errorcluster[])
      "Safety Shut Down Temp" <- w187
      "Safety Shut Down Pressure (barg)" <- w173
      "Iteration Number" <- w106
    }
    n142 = Or(x=w86, y=w94) -> (x .or. y?=w87:bool)
    n143 = node-c288(w100) -> ()  [unwired: 1 out]
  }
  n144 = call <vilib>:"DAQmx Stop Task.vi"("task/channels in"=w16, "error in"=w15) -> ("task out"=w18:refnum<k21>, "error out"=w17:errorcluster)  [unwired: 12 in]
  n145 = Index Array(array=w45, index=0) -> (element=w47:u32)
  n146 = Index Array(array=w44, index=0) -> (element=w46:errorcluster)
  n147 = call <vilib>:"DAQmx Stop Task.vi"("task/channels in"=w5, "error in"=w3) -> ("task out"=w4:refnum<k21>, "error out"=w6:errorcluster)  [unwired: 12 in]
  n148 = call <vilib>:"DAQmx Clear Task.vi"("task in"=w18, "error in"=w17) -> ()  [unwired: 13 in, 1 out]
  n149 = call <vilib>:"DAQmx Clear Task.vi"("task in"=w4, "error in"=w6) -> ()  [unwired: 13 in, 1 out]
  n150 = call "NCS_CloseDevice.vi"("error in (no error)"=w46, "device handle"=w47) -> ()  [unwired: 1 out]
  n151 = call "CN7500_Write Set Point Value.vi"("Target Set Point Value"=25, "error in (no error)"=w33, "Controller Number"=w36, "VISA In"=w32) -> ("error out"=w38:errorcluster, "VISA Out"=w39:refnum<visa-resource-name>)  [unwired: 6 in]
  n152 = call "CN7500_Close.vi"("error in (no error)"=w38, "VISA resource name"=w39) -> ()  [unwired: 9 in, 1 out]
